vi "Nanopuller_curve_selection.vi"(10 "Force curve raw":dbl[][](array[numeric]), 11 "curve selection":enum32{"approach", "retract"}(radio)) -> (3 "single FC output":dbl[][](array[numeric]))   [LabVIEW 2015]
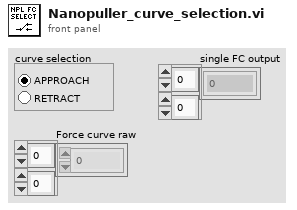
[diagram p1: front panel]
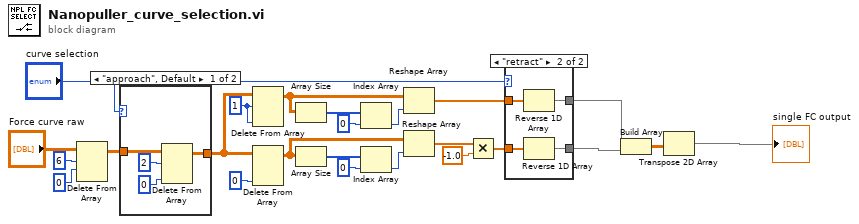
[diagram p0: block diagram]
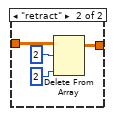
[diagram p3: hidden frame]
diagram:
  w5 = 1 ("length")
  n1 = Delete From Array(array="Force curve raw", length=6, index (row)=0 ("disabled index (col)")) -> (array with subset deleted=w4:dbl[][])  [unwired: 1 in, 1 out]
  n2 = case shown="\"approach\", Default" "curve selection" {
    tunnel: w4 -> [w26 w32]
    tunnel: [w25 w29] -> w7
    frame "approach", Default {
      n3 = Delete From Array(array=w26, length=2, index (col)=0 ("disabled index (col)")) -> (array with subset deleted=w25:dbl[][])  [unwired: 1 in, 1 out]
    }
    frame "retract" {
      n4 = Delete From Array(array=w32, length=2, index (col)=2 ("disabled index (col)")) -> (array with subset deleted=w29:dbl[][])  [unwired: 1 in, 1 out]
    }
  }
  n5 = Delete From Array(array=w7, length=w5, index (col)=w5) -> (array with subset deleted=w14:dbl[][])  [unwired: 1 in, 1 out]
  n6 = Delete From Array(array=w7, index (col)=0 ("length")) -> (array with subset deleted=w8:dbl[][])  [unwired: 2 in, 1 out]
  n7 = Array Size(array=w14) -> (size(s)=w13:i32[])
  n8 = Array Size(array=w8) -> (size(s)=w9:i32[])
  n9 = Index Array(array=w13, index=0) -> (element=w15:i32)
  n10 = Index Array(array=w9, index=0) -> (element=w11:i32)
  n11 = Reshape Array(w14, w15) -> (w22:dbl[])
  n12 = Reshape Array(w8, w11) -> (w19:dbl[])
  n13 = Multiply(x=w19, y=-1.0) -> (x*y=w21:dbl[])
  n14 = case shown="\"retract\"" "curve selection" {
    tunnel: [w34 w37] -> w24
    tunnel: w21 -> [w34 w38]
    tunnel: [w33 w35] -> w23
    tunnel: w22 -> [w33 w36]
    frame "approach", Default {
    }
    frame "retract" {
      n15 = Reverse 1D Array(array=w36) -> (reversed array=w35:dbl[])
      n16 = Reverse 1D Array(array=w38) -> (reversed array=w37:dbl[])
    }
  }
  n17 = Build Array(w23, w24) -> (w16:dbl[][])
  n18 = Transpose 2D Array(2D array=w16) -> (transposed array=→"single FC output":dbl[][])
